vi "FindLabelParams.vi"(0 "label":u32, 1 "index":i32, 5 "SDI":u8, 7 "SDI_Enabled":bool, 9 "LabelParamsArray":T1[](array[typedef]), 11 "error in":errorcluster) -> (4 "Found":bool, 6 "LabelParams":T1, 15 "error out":errorcluster)   [LabVIEW 2016]
uses:
  Controls/LabelParam.ctl
  Controls/LabelInfo.ctl
  Controls/ARINCParam.ctl
  Ballard Arinc-429 System Explorer.lvlib
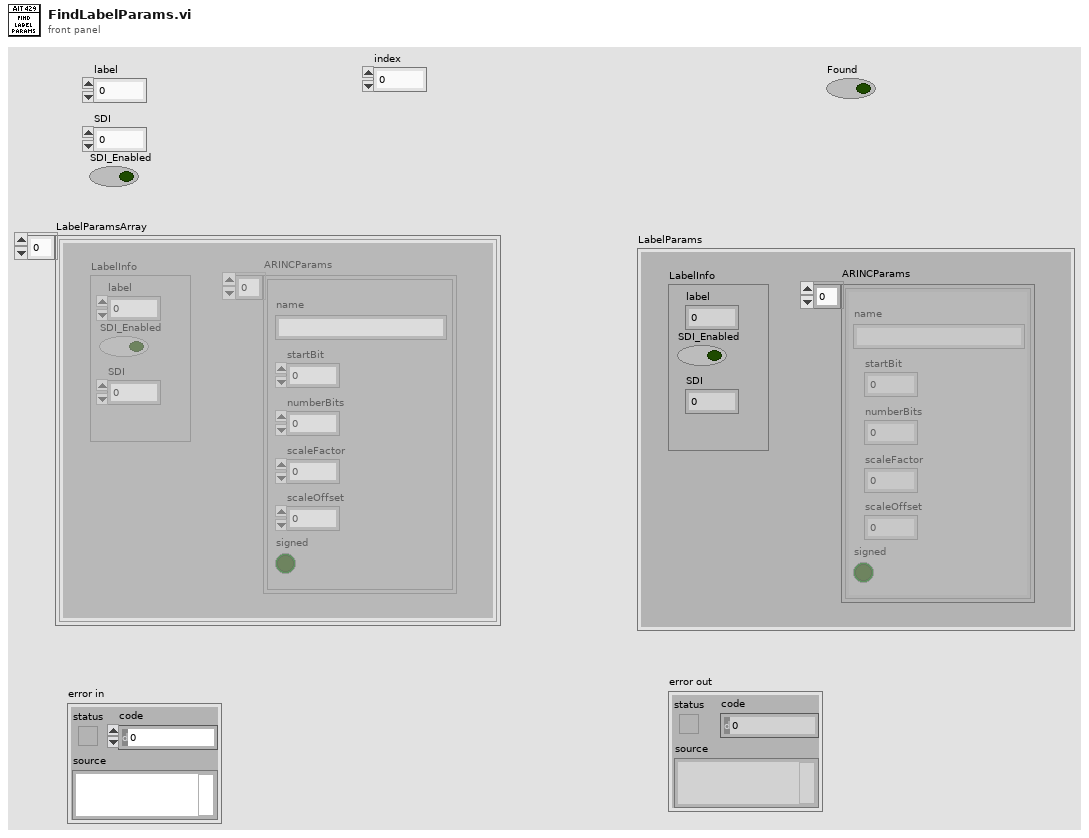
[diagram p1: front panel]
types:
  T1 = typedef "Ballard Arinc-429 System Explorer.lvlib/LabelParam.ctl" = cluster{"LabelInfo":T2, "ARINCParams":T3[]}
  T2 = typedef "Ballard Arinc-429 System Explorer.lvlib/LabelInfo.ctl" = cluster{"label":u32, "SDI_Enabled":bool, "SDI":u8}
  T3 = typedef "Ballard Arinc-429 System Explorer.lvlib/ARINCParam.ctl" = cluster{"name":string, "startBit":i32, "numberBits":i32, "scaleFactor":dbl, "scaleOffset":dbl, "signed":bool}
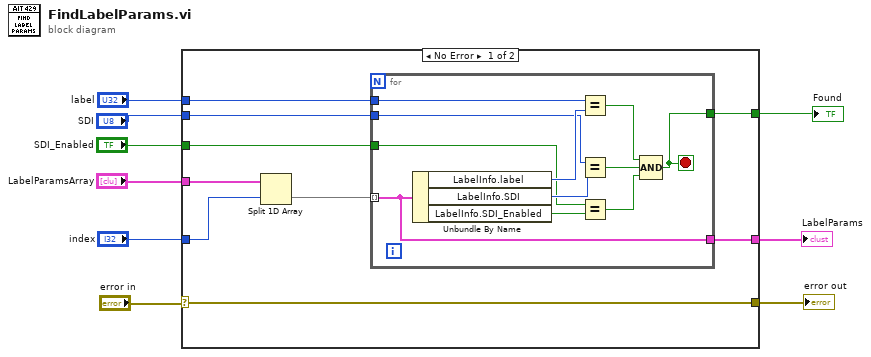
[diagram p0: block diagram]
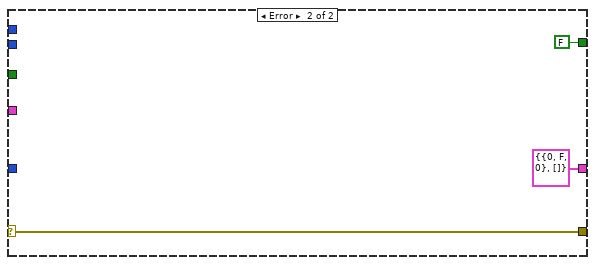
[diagram p2: hidden frame]
diagram:
  n1 = case shown="No Error" "error in" {
    selector: "error in" -> [w12 w32]
    tunnel: "index" -> [w18 _]
    tunnel: "LabelParamsArray" -> [w17 _]
    tunnel: [w15 FALSE] -> w8
    tunnel: "SDI" -> [w14 _]
    tunnel: "label" -> [w13 _]
    tunnel: [w12 w32] -> w5
    tunnel: "SDI_Enabled" -> [w11 _]
    tunnel: [w10 T1 {"LabelInfo"={"label"=0, "SDI_Enabled"=FALSE, "SDI"=0}, "ARINCParams"=[]} ("LabelParam")] -> w1
    frame No Error {
      n2 = Split 1D Array(array=w17, index=w18) -> (second subarray=w16:T1[])  [unwired: 1 out]
      n3 = for {
        tunnel: w16 -> [w19] mode=indexing
        tunnel: w13 -> [w29]
        tunnel: w14 -> [w27]
        tunnel: [w24] -> w15
        tunnel: w11 -> [w22]
        tunnel: [w19] -> w10
        stop <- w24 stop-if-true
        n4 = Unbundle By Name(w19) -> ("LabelInfo.label"=w28:u32, "LabelInfo.SDI"=w23:u8, "LabelInfo.SDI_Enabled"=w21:bool)
        n5 = Equal?(x=w29, y=w28) -> (x = y?=w26:bool)
        n6 = Equal?(x=w27, y=w23) -> (x = y?=w25:bool)
        n7 = Equal?(x=w22, y=w21) -> (x = y?=w20:bool)
        n8 = Compound Arithmetic op=AND(w26, w25, w20) -> (w24:bool)
      }
    }
    frame Error {
    }
  }
  "Found" <- w8
  "error out" <- w5
  "LabelParams" <- w1
